vi "Test - Navigating Nodes and Wires Target.vi"() -> ()   [LabVIEW 2023]
doc: "This VI serves as the target for the Navigating Nodes and Wires.vi example, which locates the One Button Dialog function in this VI and replaces the button text with \"Okay!\"\n\nDo not save changes to this VI."
panel:
  in  "message":string
  # "Select Help>>Show Context Help and move the cursor over the VI icon to display help for this VI.\n\nDO NOT SAVE CHANGES TO THIS VI. This VI serves as the target for the Navigating Nodes and Wires.vi example. Therefore, changing this VI might prevent the Navigating Nodes and Wires.vi example from demonstrating its scripting task."
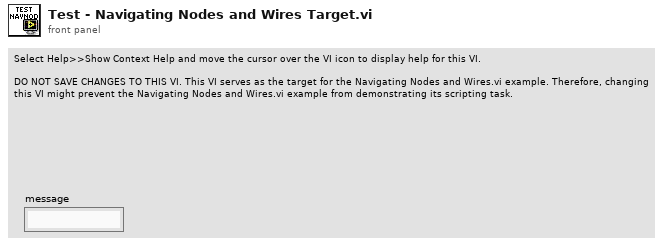
[diagram p1: front panel]
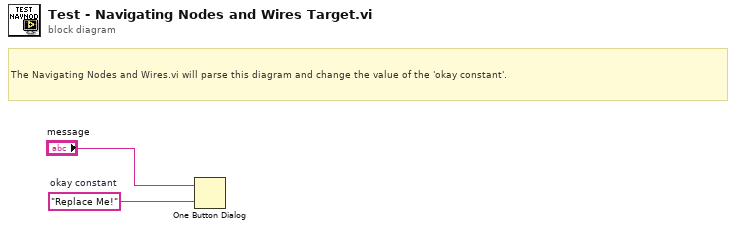
[diagram p0: block diagram]
diagram:
  w1 = "Replace Me!"  # okay constant
  # "The Navigating Nodes and Wires.vi will parse this diagram and change the value of the 'okay constant'."
  n1 = One Button Dialog(message="message", button name ("OK")=w1) -> ()  [unwired: 1 out]
